vi "IMUrollpitch.vi"(8 "Bias":T1, 9 "yAngle in":dbl, 10 "xAngle in":dbl, 11 "error in (no error)":errorcluster) -> (1 "pitch":dbl, 2 "roll":dbl, 3 "error out":errorcluster, 4 "Gyro deg/s":cluster{dbl, dbl, dbl}, 6 "Accel g's":cluster{dbl, dbl, dbl})   [LabVIEW 2016]
doc: "Inputs\nPrevious Roll\nPrevious Pitch\nBias\n\nOutput\nRoll\nPitch\n\n\nCalculates the roll and pitch angles using gyro and accelerometer values and neglects the bias values from the measurements."
uses:
  <vilib>/imath/engines/lvmath2/RunTimeEngine/BuiltInFunctions/atan2/NIMS_atan2.vi
  <instcachedir>/0/NIMS_atan2_A91AA4A7D42247EDBE8F76DB99AF04A4.lvgen/NIMS_atan2_A91AA4A7D42247EDBE8F76DB99AF04A4_000.vi
  <vilib>/imath/engines/lvmath2/RunTimeEngine/NodeEndStatement/NIMS_NodeEndStatement_Output.vi
  <instcachedir>/0/NIMS_NodeEndStatement_Output_53EC0D466D134D7ABD903AC30B43404B.lvgen/NIMS_NodeEndStatement_Output_53EC0D466D134D7ABD903AC30B43404B_001.vi
  <vilib>/imath/engines/lvmath2/RunTimeEngine/ErrorHandling/NIMS_Finalize Error.vi
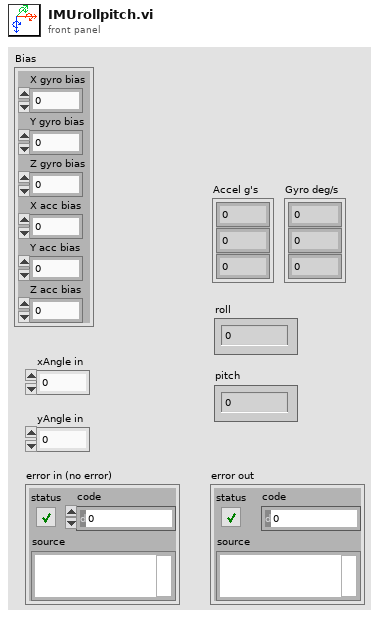
[diagram p1: front panel]
types:
  T1 = cluster{"X gyro bias":dbl, "Y gyro bias":dbl, "Z gyro bias":dbl, "X acc bias":dbl, "Y acc bias":dbl, "Z acc bias":dbl}
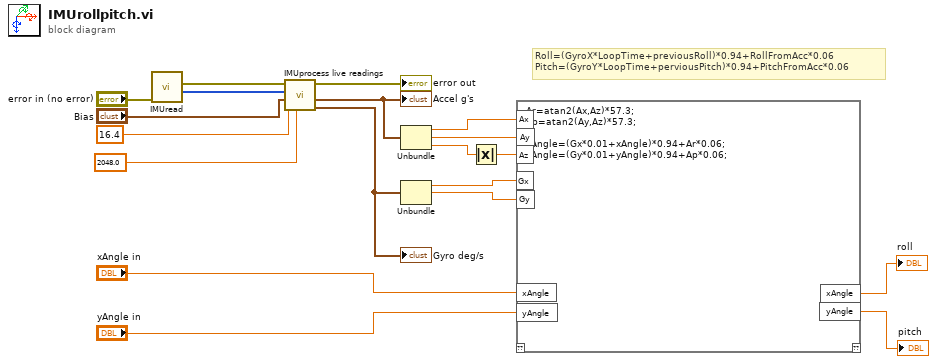
[diagram p0: block diagram]
diagram:
  # "Roll=(GyroX*LoopTime+previousRoll)*0.94+RollFromAcc*0.06\nPitch=(GyroY*LoopTime+perviousPitch)*0.94+PitchFromAcc*0.06"
  n1 = call "IMUread.vi"("error in (no error)"="error in (no error)") -> ("error out"=w10:errorcluster, "Accel, Gyro"=w5:u16[])  [unwired: 9 in]
  n2 = call "IMUprocess live readings.vi"("Acc sensivity"=2048.0 ("Acc s"), "Gyro sensivity"=16.4 ("Gyro s"), "Bias"="Bias", "Sensor Data in"=w5, "error in (no error)"=w10) -> ("Gyro deg/s"=w3:cluster{dbl, dbl, dbl}, "Accel g's"=w4:cluster{dbl, dbl, dbl}, "error out"=→"error out":errorcluster)  [unwired: 4 in]
  "Accel g's" <- w4
  "Gyro deg/s" <- w3
  n3 = Unbundle(w4) -> (w7:dbl, w8:dbl, w18:dbl)
  n4 = Unbundle(w3) -> (w9:dbl, w19:dbl)  [unwired: 1 out]
  n5 = Absolute Value(x=w18) -> (abs(x)=w17:dbl)
  n6 = mathscript code="Ar=atan2(Ax,Az)*57.3;\nAp=atan2(Ay,Az)*57.3;\n\nxAngle=(Gx*0.01+xAngle)*0.94+Ar*0.06;\nyAngle=(Gy*0.01+yAngle)*0.94+Ap*0.06;"("Ax"=w7, "Ay"=w8, "Az"=w17, "Gx"=w9, "Gy"=w19, "xAngle"="xAngle in", "yAngle"="yAngle in") -> ("xAngle"=→"roll":dbl, "yAngle"=→"pitch":dbl)  [unwired: 1 in, 1 out]
